vi "UnplanISD_Global.vi"() -> ()   [LabVIEW 2016]
doc: "-----------------------------------------------------------------------------------------------------------------------\nCopyright <2019> <The University of Tennessee at Knoxville and the University of Tennessee Research Foundation>\nThis software is released under BSD-3 \nhttps://opensource.org/licenses/BSD-3-Clause \nAdditional license options available at https://utrf.tennessee.edu/industry/sample-agreements/\n-----------------------------------------------------------------------------------------------------------------------"
panel:
  in  "Check time":bool
  in  "ISD_success":bool
  in  "Unplanned BKS":bool
  in  "Unplanned_ISD":bool
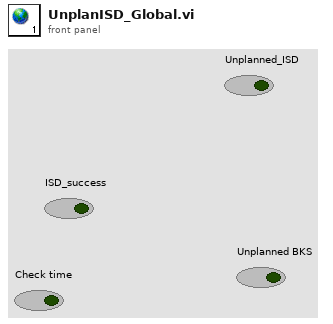
[diagram p1: front panel]
diagram:
